vi "gl_Calibration globals.vi"() -> ()   [LabVIEW 2017]
uses:
  AOL Z/Typedefs/AOL Z cal process refs.ctl
  AOL Z/Typedefs/Cal mode.ctl
  AOL Z/Typedefs/Cal points.ctl
  AOL Z/Typedefs/Cal channel.ctl
  AOL Z/Typedefs/Pre-AOL Z wizard refs.ctl
  AOL Z/Typedefs/Pockels cal process refs.ctl
panel:
  in  "FOV cal file name":string="FOV Cal.ini"
  in  "Laser power cal file name":string
  in  "Open HW channels config page":bool
  in  "Calibrating single objective":bool
  in  "Pockels cal outer loop index":i32
  in  "Objective selection index at start of Pockels cal":i32
  in  "Pockels Cal-Objective cal attempted":bool
  out "Pockels cal'd wavelengths":dbl[](array[numeric])
  in  "Laser power during pockels cal (mW)":u16
  in  "Pockels bias":i16=199
  in  "Prism 2":u16=1953
  in  "Prism 1":u16=2039
  in  "Prevent file update":bool
  in  "Pockels cal.Dwell time (µs)":dbl=0.4
  in  "Pockels cal.Zoom":u8=12
  out "Pockels Cal Window refs":cluster{"VI's reference":refnum<vi>}
  in  "Pockels cal file name":string
  in  "AOL Z cal file name":string
  in  "Pockels ctrl V for cal process":dbl min=-1.0 max=1.0 step=0.1
  out "Pockels cal process refs":T1
  in  "Pockels Cal wizard is running":bool
  in  "Pockels Cal window is open":bool
  in  "Pockels Cal-Bring to front":bool
  in  "Wizard window refs":T2
  in  "Channel Selector":T3
  in  "Calibration points":T4=enum."21-points calibration"
  in  "Display message":string
  in  "Calibration Mode":T5
  in  "Base string":string
  out "AOL Z cal process refs":T6
  in  "AOL Cal wizard is running":bool
  in  "AOL-Z Cal window is open":bool
  in  "Norm coord for cal process":dbl min=-1.0 max=1.0 step=0.1
  out "Motor Z Cal Window refs":cluster{"VI's reference":refnum<vi>}
  in  "AOL-Z Cal-Bring to front":bool
  # "AOL Z Calibration globals"
  # "Laser Power Calibration globals"
  # "Pockels Calibration globals"
  # "FOV Calibration globals"
  # "Common calibration globals"
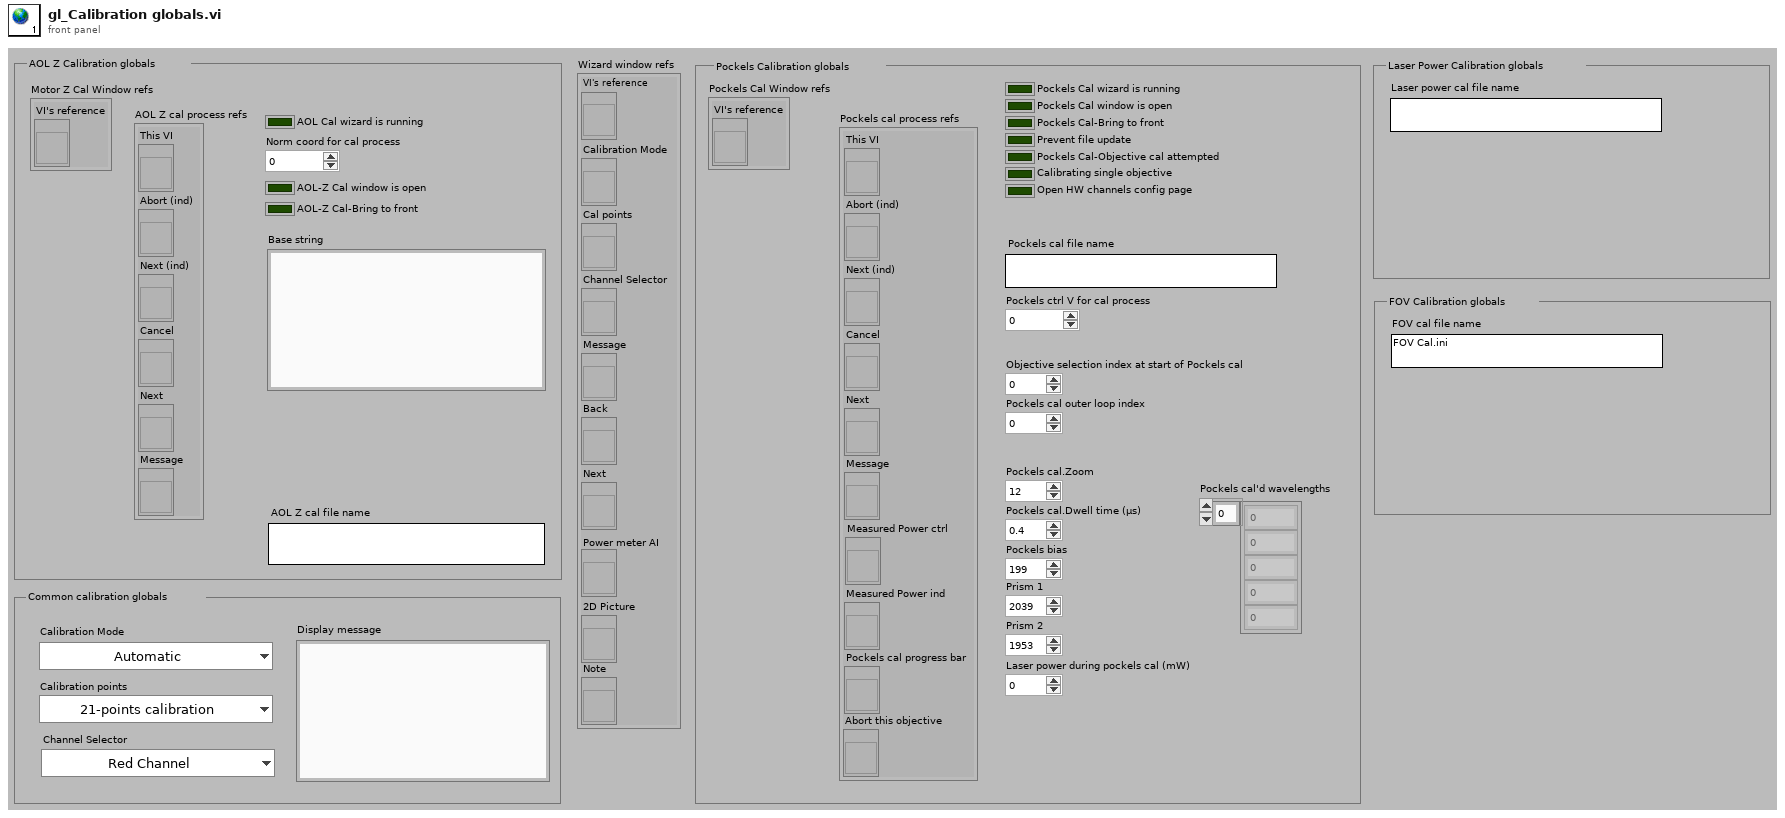
[diagram p1: front panel]
types:
  T1 = typedef "Pockels cal process refs.ctl" = cluster{"This VI":refnum<vi>, "Abort (ind)":refnum<vi>, "Next (ind)":refnum<vi>, "Cancel":refnum<vi>, "Next":refnum<vi>, "Message":refnum<vi>, "Measured Power ctrl":refnum<vi>, "Measured Power ind":refnum<vi>, "Pockels cal progress bar":refnum<vi>, "Abort this objective":refnum<vi>}
  T2 = typedef "Pre-AOL Z wizard refs.ctl" = cluster{"VI's reference":refnum<vi>, "Calibration Mode":refnum<vi>, "Cal points":refnum<vi>, "Channel Selector":refnum<vi>, "Message":refnum<vi>, "Back":refnum<vi>, "Next":refnum<vi>, "Power meter AI":refnum<vi>, "2D Picture":refnum<vi>, "Note":refnum<vi>}
  T3 = typedef "Cal channel.ctl" = enum16{"Red Channel", "Green Channel"}
  T4 = typedef "Cal points.ctl" = enum16{"5-points calibration (crude)", "11-points calibration", "21-points calibration", "41-points calibration"}
  T5 = typedef "Cal mode.ctl" = enum16{"Automatic", "Interactive"}
  T6 = typedef "AOL Z cal process refs.ctl" = cluster{"This VI":refnum<vi>, "Abort (ind)":refnum<vi>, "Next (ind)":refnum<vi>, "Cancel":refnum<vi>, "Next":refnum<vi>, "Message":refnum<vi>}
diagram:
